vi "Send Pedigree.vi"(8 "error in":errorcluster, 10 "Pedigree":enum16{"STAT", "BB", "PT", "EM", "FT"}(ring), 11 "Engine in":refnum<class "Engine.lvclass">) -> (0 "error out":errorcluster, 3 "Engine out":refnum<class "Engine.lvclass">)   [LabVIEW 2023, in "Engine.lvlib" / "Engine.lvclass"]
doc: "Trigger the Update Pedigree Event (allowing components to update any references to the Pedigree)"
uses:
  Project/Engine.lvclass
  Project/Engine.lvclass/Engine.ctl
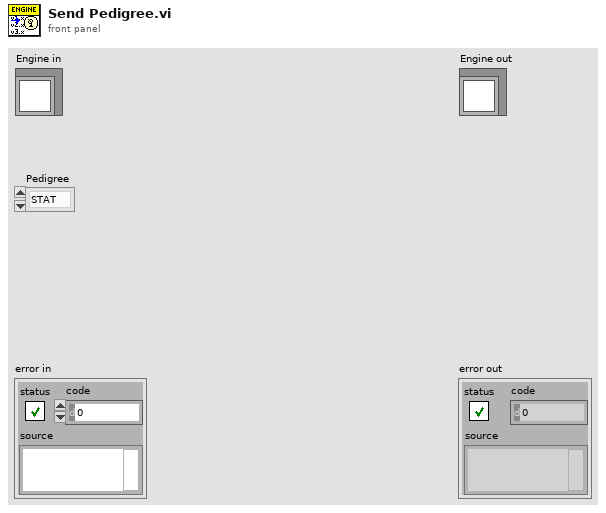
[diagram p1: front panel]
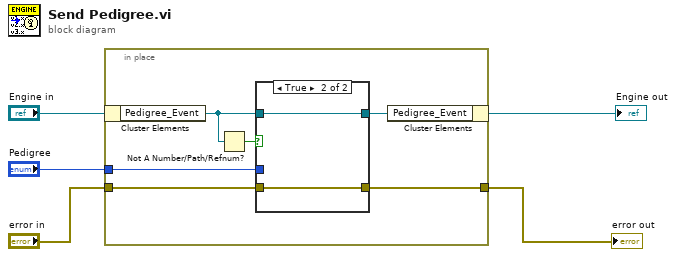
[diagram p0: block diagram]
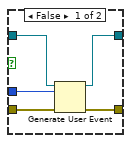
[diagram p2: hidden frame]
diagram:
  n1 = in-place {
    in-place-border: "error in" -> [w10]
    in-place-border: [w9] -> w2
    in-place-border: "Pedigree" -> [w8]
    n2 = in-place-cluster #1("Engine in") -> ("Pedigree_Event"=w7:refnum<user-event>)
    n3 = Not A Number/Path/Refnum?(number/path/refnum=w7) -> (NaN/Path/Refnum?=w6:bool)
    n4 = case shown="True" w6 {
      tunnel: [w16 w18] -> w11
      tunnel: w10 -> [w15 w17]
      tunnel: [w14 w17] -> w9
      tunnel: w8 -> [w13 _]
      tunnel: w7 -> [w12 w18]
      frame False {
        n5 = Generate User Event(user event=w12, event data cluster=w13, error in=w15) -> (user event out=w16:refnum<user-event>, error out=w14:errorcluster)  [unwired: 1 in]
      }
      frame True {
      }
    }
    n6 = in-place-cluster #1("Pedigree_Event"=w11) -> (→"Engine out":refnum<class "Engine.lvclass">)
  }
  "error out" <- w2
